vi "expression_to_string.vi"(6 "ShowType?":bool, 8 "error in (no error)":errorcluster, 11 "Expression":T1) -> (0 "error out":errorcluster, 3 "String":string)   [LabVIEW 2021]
uses:
  Expression.ctl
  ExpressionType.ctl
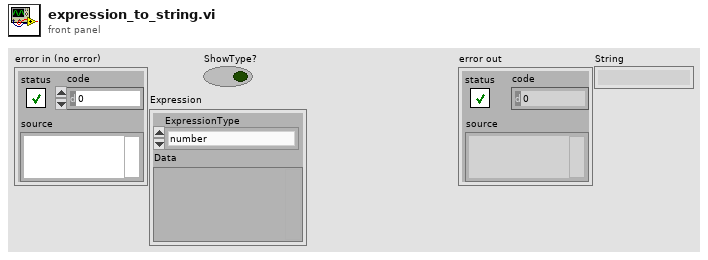
[diagram p1: front panel]
types:
  T1 = typedef "Expression.ctl" = cluster{"ExpressionType":T2, "Data":variant}
  T2 = typedef "ExpressionType.ctl" = enum16{"number", "string", "symbol", "primitive", "list", "closure", "nil", "error"}
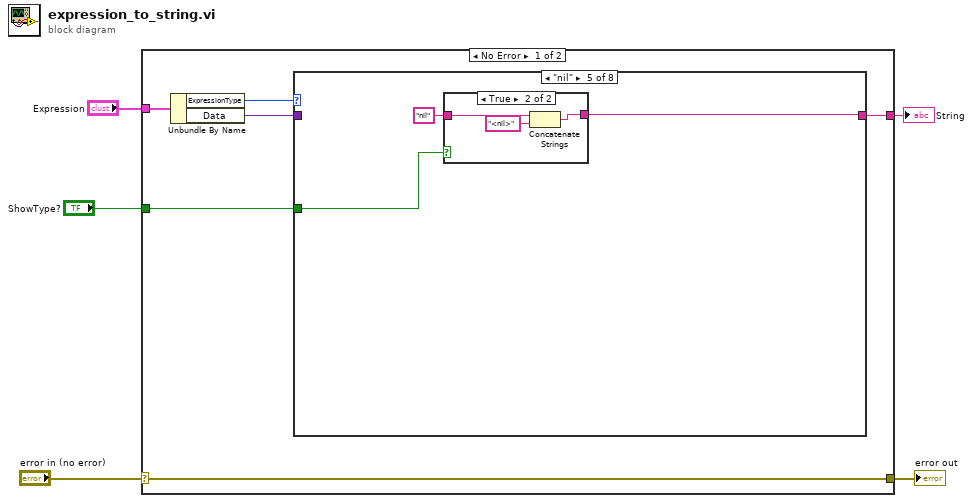
[diagram p0: block diagram]
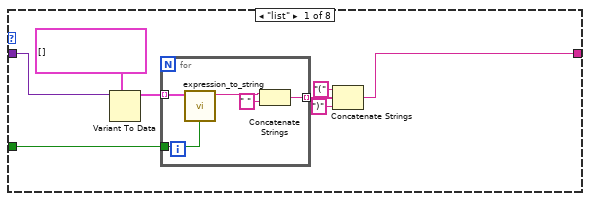
[diagram p2: hidden frame]
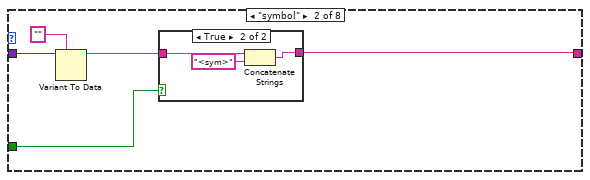
[diagram p3: hidden frame]
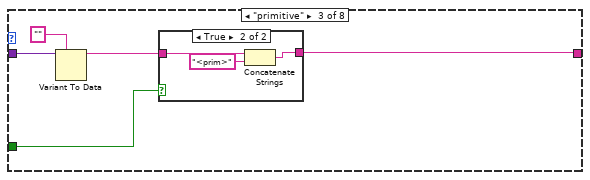
[diagram p5: hidden frame]
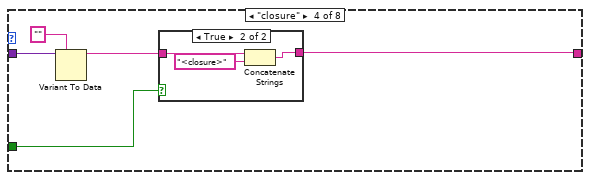
[diagram p7: hidden frame]
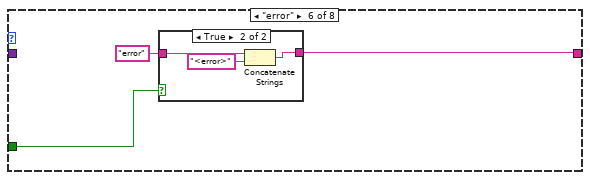
[diagram p10: hidden frame]
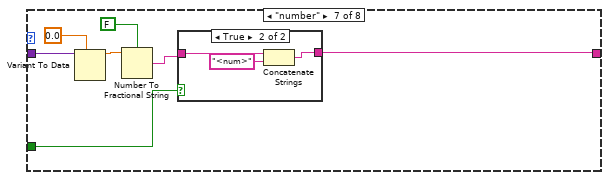
[diagram p12: hidden frame]
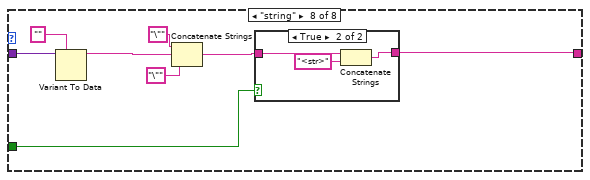
[diagram p14: hidden frame]
diagram:
  n1 = case shown="No Error" "error in (no error)" {
    selector: "error in (no error)" -> [w11 w89]
    tunnel: [w11 w89] -> w4
    tunnel: "Expression" -> [w10 _]
    tunnel: [w7 _] -> w3
    tunnel: "ShowType?" -> [w6 _]
    frame No Error {
      n2 = Unbundle By Name(w10) -> ("ExpressionType"=w9:T2, "Data"=w8:variant)
      n3 = case shown="\"nil\"" w9 {
        tunnel: w8 -> [w19 w29 w38 w47 _ _ w72 w84]
        tunnel: [w14 w26 w35 w44 w54 w61 w71 w81] -> w7
        tunnel: w6 -> [w13 w25 w34 w43 w53 w60 w70 w82]
        frame "list" {
          n4 = Variant To Data(type=T1[] [], Variant=w19) -> (data=w18:T1[])  [unwired: 1 in, 1 out]
          n5 = for {
            tunnel: w18 -> [w22] mode=indexing
            tunnel: [w23] -> w17 mode=indexing
            tunnel: w13 -> [w21]
            n6 = call "expression_to_string.vi"("ShowType?"=w21, "Expression"=w22) -> ("String"=w20:string)  [unwired: 8 in, 1 out]
            n7 = Concatenate Strings(w20, " " ("string")) -> (w23:string)
          }
          n8 = Concatenate Strings("(" ("string"), w17, ")" ("string")) -> (w14:string)
        }
        frame "symbol" {
          n9 = Variant To Data(type="", Variant=w29) -> (data=w27:string)  [unwired: 1 in, 1 out]
          n10 = case shown="True" w25 {
            tunnel: [w30 w32] -> w26
            tunnel: w27 -> [w30 w33]
            frame False {
            }
            frame True {
              n11 = Concatenate Strings(w33, "<sym>" ("string")) -> (w32:string)
            }
          }
        }
        frame "primitive" {
          n12 = Variant To Data(type="", Variant=w38) -> (data=w36:string)  [unwired: 1 in, 1 out]
          n13 = case shown="True" w34 {
            tunnel: [w39 w41] -> w35
            tunnel: w36 -> [w39 w42]
            frame False {
            }
            frame True {
              n14 = Concatenate Strings(w42, "<prim>" ("string")) -> (w41:string)
            }
          }
        }
        frame "closure" {
          n15 = Variant To Data(type="", Variant=w47) -> (data=w45:string)  [unwired: 1 in, 1 out]
          n16 = case shown="True" w43 {
            tunnel: [w48 w50] -> w44
            tunnel: w45 -> [w48 w51]
            frame False {
            }
            frame True {
              n17 = Concatenate Strings(w51, "<closure>" ("string")) -> (w50:string)
            }
          }
        }
        frame "nil" {
          n18 = case shown="True" w53 {
            tunnel: [w55 w57] -> w54
            tunnel: "nil" -> [w55 w58]
            frame False {
            }
            frame True {
              n19 = Concatenate Strings(w58, "<nil>" ("string")) -> (w57:string)
            }
          }
        }
        frame "error" {
          n20 = case shown="True" w60 {
            tunnel: [w62 w64] -> w61
            tunnel: "error" -> [w62 w65]
            frame False {
            }
            frame True {
              n21 = Concatenate Strings(w65, "<error>" ("string")) -> (w64:string)
            }
          }
        }
        frame "number" {
          n22 = Variant To Data(type=0.0, Variant=w72) -> (data=w68:dbl)  [unwired: 1 in, 1 out]
          n23 = Number To Fractional String(use system decimal point (T)=FALSE, number=w68) -> (F-format string=w67:string)  [unwired: 2 in]
          n24 = case shown="True" w70 {
            tunnel: [w73 w75] -> w71
            tunnel: w67 -> [w73 w76]
            frame False {
            }
            frame True {
              n25 = Concatenate Strings(w76, "<num>" ("string")) -> (w75:string)
            }
          }
        }
        frame "string" {
          n26 = Variant To Data(type="", Variant=w84) -> (data=w78:string)  [unwired: 1 in, 1 out]
          n27 = Concatenate Strings("\"" ("string"), w78, "\"" ("string")) -> (w77:string)
          n28 = case shown="True" w82 {
            tunnel: [w85 w87] -> w81
            tunnel: w77 -> [w85 w88]
            frame False {
            }
            frame True {
              n29 = Concatenate Strings(w88, "<str>" ("string")) -> (w87:string)
            }
          }
        }
      }
    }
    frame Error {
      # "Wire the error cluster across even in the \"No Error\"\ncase so that warnings get propagated."
    }
  }
  "error out" <- w4
  "String" <- w3
